vi "SetAppData.vi"(8 "Error In":errorcluster[](array[cluster]), 9 "XmlData":string, 10 "arg":string, 11 "Bus in":refnum<class "Bus.lvclass">) -> (0 "Error Out":errorcluster[](array[cluster]), 3 "Bus out":refnum<class "Bus.lvclass">)   [LabVIEW 2017, in "Bus_class.lvlib" / "Bus.lvclass"]
uses:
  Bus.lvclass
  Bus.lvclass/Bus.ctl
  <vilib>/Utility/error.llb/Error Cluster From Error Code.vi
  <vilib>/ErrorRing/Error Ring.xnode
  <userlib>/NIST/NISTErrorLib/NISTErrorLib.lvlib
  Modules/AppModule/AppModule.lvlib
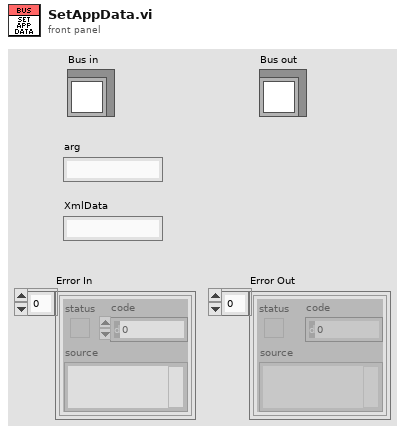
[diagram p1: front panel]
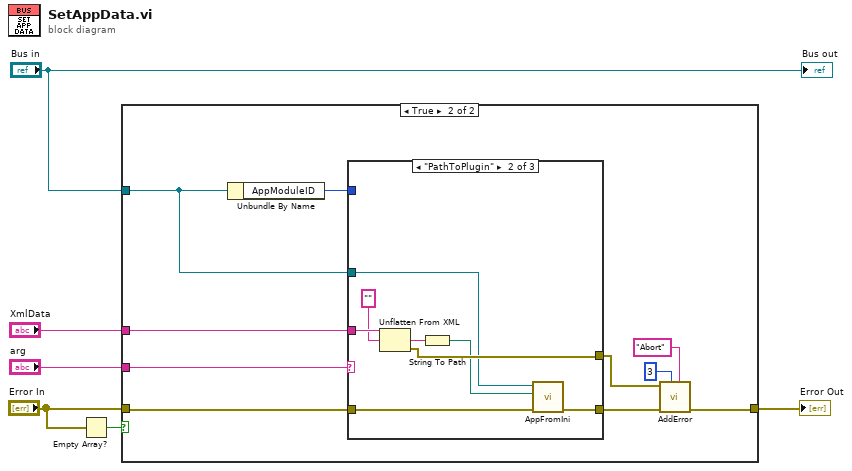
[diagram p0: block diagram]
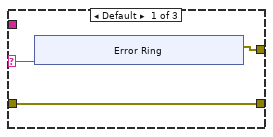
[diagram p3: hidden frame]
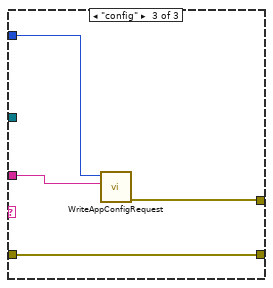
[diagram p4: hidden frame]
diagram:
  n1 = Empty Array?(array="Error In") -> (empty?=w6:bool)
  n2 = case shown="True" w6 {
    tunnel: "Error In" -> [w7 w8]
    tunnel: [w7 w17] -> w4
    tunnel: "Bus in" -> [_ w9]
    tunnel: "arg" -> [_ w16]
    tunnel: "XmlData" -> [_ w15]
    frame False {
    }
    frame True {
      n3 = Unbundle By Name(w9) -> ("AppModuleID"=w14:i32)
      n4 = case shown="\"PathToPlugin\"" w16 {
        selector: w16 -> [w20 _ _]
        tunnel: w14 -> [_ _ w39]
        tunnel: w15 -> [_ w35 w37]
        tunnel: [w19 w30 w38] -> w11
        tunnel: w8 -> [w18 w32 w36]
        tunnel: [w18 w31 w36] -> w10
        tunnel: w9 -> [_ w28 _]
        frame Default {
          n5 = xnode "Error Ring"("parameter 0"=w20) -> ("error out"=w19:errorcluster)
        }
        frame "PathToPlugin" {
          n6 = Unflatten From XML(xml string=w35, type="") -> (value=w33:string, error out=w30:errorcluster)  [unwired: 1 in]
          n7 = String To Path(string=w33) -> (path=w29:path)
          n8 = call "AppFromIni.vi"("ErrorArray In"=w32, "PathToIni"=w29, "Bus in"=w28) -> ("ErrorArray Out"=w31:errorcluster[])  [unwired: 7 in, 1 out]
        }
        frame "config" {
          n9 = call "WriteAppConfigRequest.vi"("AppConfigXML"=w37, "ModuleID"=w39) -> ("error out"=w38:errorcluster)  [unwired: 9 in]
        }
      }
      n10 = call <userlib>:"AddError.vi"("Severity"="Abort", "Priority"=u8 3, "ErrorArray"=w10, "error in (no error)"=w11) -> ("ErrorArray"=w17:errorcluster[])  [unwired: 6 in, 1 out]
    }
  }
  "Error Out" <- w4
  "Bus out" <- "Bus in"
